vi "Configure Channels.vi"(8 "error in (no error)":errorcluster, 11 "Fetch Waveform CFG in":refnum<class "Thermometer DAQmx Config.lvclass">) -> (0 "error out":errorcluster, 3 "Fetch Waveform CFG out":refnum<class "Thermometer DAQmx Config.lvclass">)   [LabVIEW 2023, in "Thermometer.lvlib" / "Thermometer DAQmx.lvlib" / "Thermometer DAQmx Config.lvclass"]
uses:
  Thermometer DAQmx Config.lvclass
  Configuration Base/Configuration Base.lvclass/Configuration Base.ctl
  Thermometer DAQmx Config.lvclass/Thermometer DAQmx Config.ctl
  2bbd9918-bd9c-41c6-ab27-318135d6589f.vi
  7bb3278f-f317-49b8-b679-350ee40640c1.vi
  9ef34f08-4c6e-4249-b0b4-5be22f06c902.vi
  3b398603-2ca1-435f-b72b-9f06b97abd3e.vi
  8c67670f-e3d6-4b33-b541-3e0c066aa62d.vi
  e6615cb0-8fb3-414a-9750-8123ab60430d.vi
  e76095fd-35b4-4b09-aa72-0d6101ce3055.vi
  1c43d64f-8910-4a04-aaaa-8e70328cfd49.vi
  <vilib>/JDP Science/JSONtext/Next JSON Value.vi
  <vilib>/JDP Science/JSONtext/String Subset.vi
  <vilib>/JDP Science/JSONtext/Parsing/Advance past next JSON Value (inlined COPY).vi
  <vilib>/JDP Science/JSONtext/Parsing/Advance past whitespace.vi
  <vilib>/JDP Science/JSONtext/Parsing/Advance past String.vi
  <vilib>/JDP Science/JSONtext/Parsing/Advance past Number.vi
  <vilib>/JDP Science/JSONtext/Parsing/Advance past Line Ending.vi
  <vilib>/JDP Science/JSONtext/Parsing/Parse Full Path or Item Name.vi
  <vilib>/JDP Science/JSONtext/Parsing/Advance past Array.vi
  <vilib>/JDP Science/JSONtext/Parsing/Advance past Object.vi
  <vilib>/JDP Science/JSONtext/support/Error Cluster From Code.vi
  <vilib>/JDP Science/JSONtext/Offset/Find Item Locations by Path.vi
  <vilib>/JDP Science/JSONtext/JSON text to Variant.vi
  <vilib>/Utility/error.llb/Error Cluster From Error Code.vi
  <vilib>/DAQmx/create/channels.llb/DAQmx Create Channel (AI-Temperature-Thermocouple).vi
  <vilib>/JDP Science/JSONtext/LVClass Serializer/JSONtext LVClass Serializer.lvclass
  <vilib>/ErrorRing/Error Ring.xnode
  Configuration Base/Configuration Base.lvclass
  <resource>/objmgr/daqmx.rc
  <vilib>/JDP Science/JSONtext/JSONtext.lvlib
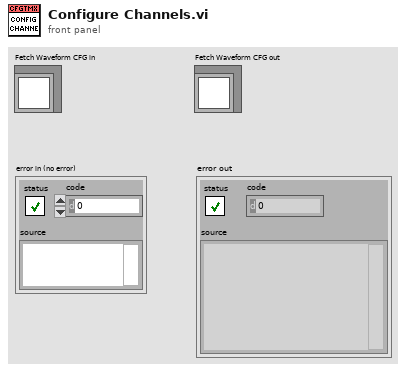
[diagram p1: front panel]
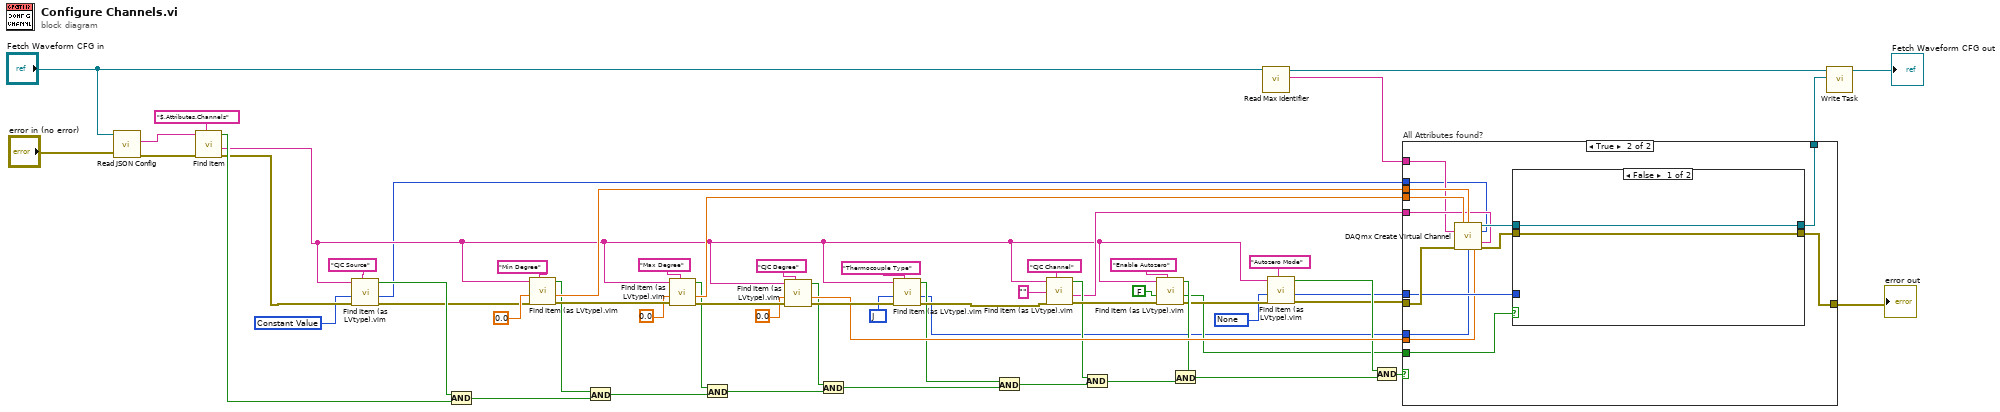
[diagram p0: block diagram]
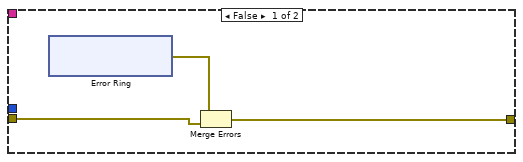
[diagram p2: hidden frame]
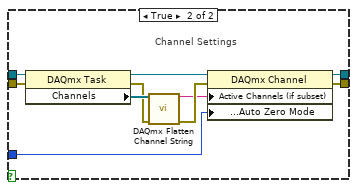
[diagram p3: hidden frame]
diagram:
  w2 = 10230 items=["None"=10230, "Once"=10244, "Every Sample"=10164] ("AI.AutoZeroMode")
  w1 = 10072 items=["J"=10072, "K"=10073, "N"=10077, "R"=10082, "S"=10085, "T"=10086, "B"=10047, "E"=10055] ("thermocouple type")
  w3 = 10116 items=["Built-In"=10200, "Constant Value"=10116, "Channel"=10113] ("cjc source")
  n1 = call "Read JSON Config.vi"("error in"="error in (no error)", "object in"="Fetch Waveform CFG in") -> ("error out"=w61:errorcluster, "<JSON>Config"=w59:string)  [unwired: 7 in, 1 out]
  n2 = call <vilib>:"Find Item.vi"("$Path or Item Name"="$.Attributes.Channels", "error in (no error)"=w61, "JSON"=w59) -> ("error out"=w9:errorcluster, "<JSON>"=w10:string, "Found"=w60:bool)  [unwired: 5 in, 1 out]
  n3 = call "Find Item (as LVtype).vim"("$Path or Item Name"="CJC Source", "error in (no error)"=w9, "Data Type and Default Value"=w3, "JSON"=w10) -> ("error out"=w7:errorcluster, "Data"=w8:i32, "Found"=w33:bool)  [unwired: 4 in, 1 out]
  n4 = And(x=w33, y=w60) -> (x .and. y?=w31:bool)
  n5 = call "Find Item (as LVtype).vim"("$Path or Item Name"="Min Degree", "error in (no error)"=w7, "Data Type and Default Value"=0.0, "JSON"=w10) -> ("error out"=w49:errorcluster, "Data"=w42:dbl, "Found"=w32:bool)  [unwired: 4 in, 1 out]
  n6 = And(x=w32, y=w31) -> (x .and. y?=w29:bool)
  n7 = call "Find Item (as LVtype).vim"("$Path or Item Name"="Max Degree", "error in (no error)"=w49, "Data Type and Default Value"=0.0, "JSON"=w10) -> ("error out"=w46:errorcluster, "Data"=w41:dbl, "Found"=w30:bool)  [unwired: 4 in, 1 out]
  n8 = And(x=w30, y=w29) -> (x .and. y?=w27:bool)
  n9 = call "Find Item (as LVtype).vim"("$Path or Item Name"="CJC Degree", "error in (no error)"=w46, "Data Type and Default Value"=0.0, "JSON"=w10) -> ("error out"=w43:errorcluster, "Data"=w40:dbl, "Found"=w28:bool)  [unwired: 4 in, 1 out]
  n10 = And(x=w28, y=w27) -> (x .and. y?=w25:bool)
  n11 = call "Find Item (as LVtype).vim"("$Path or Item Name"="Thermocouple Type", "error in (no error)"=w43, "Data Type and Default Value"=w1, "JSON"=w10) -> ("error out"=w38:errorcluster, "Data"=w6:i32, "Found"=w26:bool)  [unwired: 4 in, 1 out]
  n12 = And(x=w26, y=w25) -> (x .and. y?=w23:bool)
  n13 = call "Find Item (as LVtype).vim"("$Path or Item Name"="CJC Channel", "error in (no error)"=w38, "Data Type and Default Value"="" ("CJC Channel"), "JSON"=w10) -> ("error out"=w37:errorcluster, "Data"=w11:string, "Found"=w24:bool)  [unwired: 4 in, 1 out]
  n14 = And(x=w24, y=w23) -> (x .and. y?=w21:bool)
  n15 = call "Find Item (as LVtype).vim"("$Path or Item Name"="Enable Autozero", "error in (no error)"=w37, "Data Type and Default Value"=FALSE, "JSON"=w10) -> ("error out"=w20:errorcluster, "Data"=w15:bool, "Found"=w22:bool)  [unwired: 4 in, 1 out]
  n16 = And(x=w22, y=w21) -> (x .and. y?=w14:bool)
  n17 = call "Read Max Identifier.vi"("Thermometer DAQmx Config in"="Fetch Waveform CFG in") -> ("Max Identifier"=w51:string, "Thermometer DAQmx Config out"=w54:refnum<class "Thermometer DAQmx Config.lvclass">)  [unwired: 8 in, 1 out]
  n18 = call "Find Item (as LVtype).vim"("$Path or Item Name"="Autozero Mode", "error in (no error)"=w20, "Data Type and Default Value"=w2, "JSON"=w10) -> ("error out"=w5:errorcluster, "Data"=w4:i32, "Found"=w17:bool)  [unwired: 4 in, 1 out]
  n19 = And(x=w17, y=w14) -> (x .and. y?=w18:bool)
  n20 = case "All Attributes found?" shown="True" w18 {
    tunnel: w8 -> [_ w71]
    tunnel: w42 -> [_ w82]
    tunnel: w41 -> [_ w81]
    tunnel: w5 -> [w62 w80]
    tunnel: w40 -> [_ w74]
    tunnel: w6 -> [_ w70]
    tunnel: [w63 w78] -> w56
    tunnel: w51 -> [_ w72]
    tunnel: [_ w77] -> w53
    tunnel: w4 -> [_ w76]
    tunnel: w15 -> [_ w75]
    tunnel: w11 -> [_ w73]
    frame False {
      n21 = xnode "Error Ring"() -> ("error out"=w64:errorcluster)
      n22 = Merge Errors(w64, w62) -> (w63:errorcluster)
    }
    frame True {
      n23 = call-poly <vilib>:"DAQmx Create Virtual Channel.vi"("maximum value"=w81, "minimum value"=w82, "physical channels"=w72, "cjc source"=w71, "cjc channel"=w73, "error in"=w80, "thermocouple type"=w70, "cjc value"=w74) -> ("task out"=w83:refnum<k21>, "error out"=w79:errorcluster)  [unwired: 6 in]
      n24 = case shown="False" w75 {
        tunnel: w83 -> [w84 w95]
        tunnel: w79 -> [w85 w89]
        tunnel: [w85 w88] -> w78
        tunnel: [w84 w87] -> w77
        tunnel: w76 -> [_ w86]
        frame False {
        }
        frame True {
          # "Channel Settings"
          n25 = property class="DAQmx Task"(reference=w95, error in=w89) -> (reference out=w93:refnum<k21>, error out=w91:errorcluster, "Channels"=w94:refnum<k21>[])
          n26 = call <vilib>:"DAQmx Flatten Channel String.vi"("names in"=w94, "error in"=w91) -> ("names out"=w90:string, "error out"=w92:errorcluster)  [unwired: 12 in]
          n27 = property class="DAQmx Channel"(reference=w93, error in=w92, "Active Channels (if subset)"=w90, "Analog Input:General Properties:Advanced:High Accuracy Settings:Auto Zero Mode"=w86) -> (reference out=w87:refnum<k21>, error out=w88:errorcluster)
        }
      }
    }
  }
  "error out" <- w56
  n28 = call "Write Task.vi"("Task"=w53, "Thermometer DAQmx Config in"=w54) -> ("Thermometer DAQmx Config out"=→"Fetch Waveform CFG out":refnum<class "Thermometer DAQmx Config.lvclass">)  [unwired: 8 in, 1 out]
